vi "Setoutput.vi"(8 "error in (no error)":errorcluster, 10 "enable":bool, 11 "B&K Precision 9120 series in":refnum<class "B&K Precision 9120 series.lvclass">) -> (0 "error out":errorcluster, 2 "actual_state":bool, 3 "B&K Precision 9120 series out":refnum<class "B&K Precision 9120 series.lvclass">)   [LabVIEW 2014, in "B&K Precision 9120 series.lvclass"]
uses:
  B&K Precision 9120 series.lvclass
  B&K Precision 9120 series.lvclass/B&K Precision 9120 series.ctl
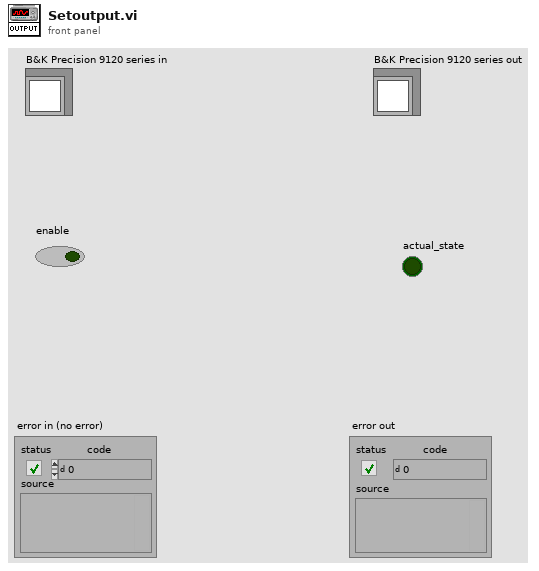
[diagram p1: front panel]
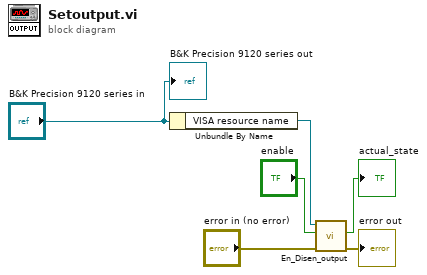
[diagram p0: block diagram]
diagram:
  n1 = Unbundle By Name("B&K Precision 9120 series in") -> ("VISA resource name"=w4:refnum<visa-resource-name>)
  n2 = call "En_Disen_output.vi"("error in (no error)"="error in (no error)", "newstate"="enable", "VISA resource in"=w4) -> ("error out"=→"error out":errorcluster, "actual_state"=→"actual_state":bool)  [unwired: 6 in, 1 out]
  "B&K Precision 9120 series out" <- "B&K Precision 9120 series in"
